vi "Handle Error.vi"(8 "error in (no error)":errorcluster, 11 "WebSocket in":refnum<class "WebSocket.lvclass">) -> (0 "error out":errorcluster, 2 "stop actor?":bool=TRUE, 3 "WebSocket out":refnum<class "WebSocket.lvclass">)   [LabVIEW 2019, in "WebSocket.lvlib" / "WebSocket.lvclass"]
doc: "(<B>Filename</B>: Actor Framework.lvlib:Actor.lvclass:Handle Error.vi)\n\nDefines how the actor handles an error that occurred while processing a message. By default, this method does nothing except stop the actor."
uses:
  WebSocket.lvclass
  C:/Program Files/National Instruments/LabVIEW 2019/vi.lib/ActorFramework/Actor/Actor.lvclass
  <vilib>/ActorFramework/Actor/Actor.lvclass/Actor.ctl
  <vilib>/ActorFramework/Message Enqueuer/Message Enqueuer.lvclass/Message Enqueuer.ctl
  <vilib>/ActorFramework/Message Enqueuer/Init from Existing Queue.vi
  <vilib>/ActorFramework/Message Enqueuer/Enqueue.vi
  WebSocket Messages/WaitListener Msg/WaitListener Msg.lvclass
  C:/Program Files/National Instruments/LabVIEW 2019/vi.lib/ActorFramework/Message/Message.lvclass
  <vilib>/ActorFramework/Message Priority Queue/Priority Enqueue.vi
  <vilib>/ActorFramework/Message Enqueuer/Message Enqueuer.lvclass
  <vilib>/ActorFramework/Actor/Actor.lvclass
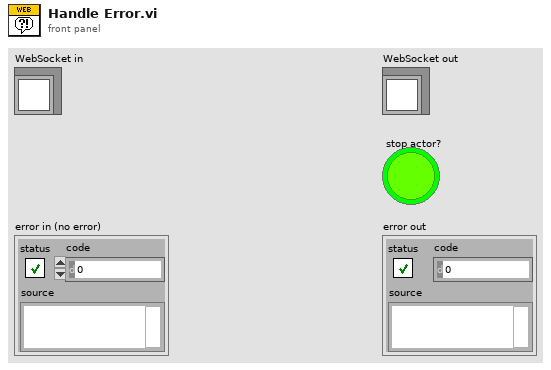
[diagram p1: front panel]
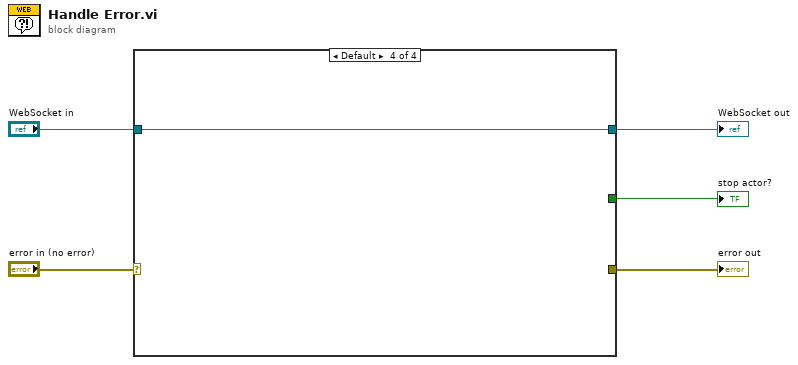
[diagram p0: block diagram]
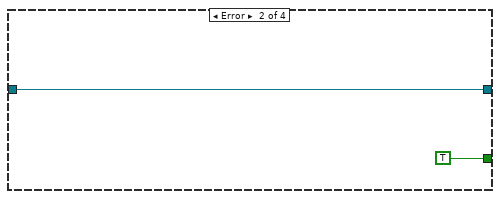
[diagram p3: hidden frame]
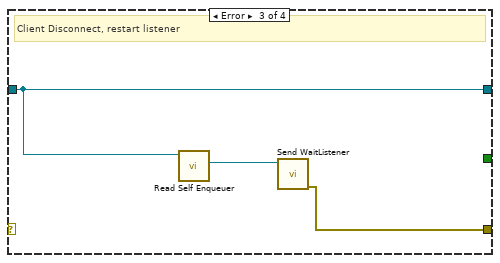
[diagram p4: hidden frame]
diagram:
  n1 = case shown="Default" "error in (no error)" {
    selector: "error in (no error)" -> [w6 _ _ _]
    tunnel: [_ TRUE _ _] -> w4
    tunnel: "WebSocket in" -> [w7 w8 w12 w13]
    tunnel: [w7 w8 w12 w13] -> w2
    tunnel: [w6 _ w10 _] -> w1
    frame No Error {
    }
    frame Error {
    }
    frame Error {
      # "Client Disconnect, restart listener"
      n2 = call <vilib>:"Read Self Enqueuer.vi"("Actor"=w12) -> ("Self Enqueuer"=w11:refnum<class "Message Enqueuer.lvclass">)  [unwired: 10 in]
      n3 = call "Send WaitListener.vi"("Message Enqueuer"=w11) -> ("error out"=w10:errorcluster)  [unwired: 9 in, 1 out]
    }
    frame Default {
    }
  }
  "WebSocket out" <- w2
  "error out" <- w1
  "stop actor?" <- w4
